vi "ComputeAreaUsingMoment.vi"(10 "Image In":T1) -> (1 "w_fy":dbl, 2 "w_fx":dbl, 4 "Y Centroid":sgl, 5 "X Centroid":sgl)   [LabVIEW 2018]
uses:
  <vilib>/vision/Image Controls.llb/IMAQ Image.ctl
  <vilib>/vision/NI_Vision_Development_Module.lvlib
panel:
  in  "File Path":path
  out "<xy>":dbl
  out "E(x,y)(x-xbar)(y-ybar)":dbl
  out "<y^2>":dbl
  out "E(x,y)(y-ybar)^2":dbl
  out "<x^2>":dbl
  out "E(x,y)(x-xbar)^2":dbl
  out "E(x,y)":dbl
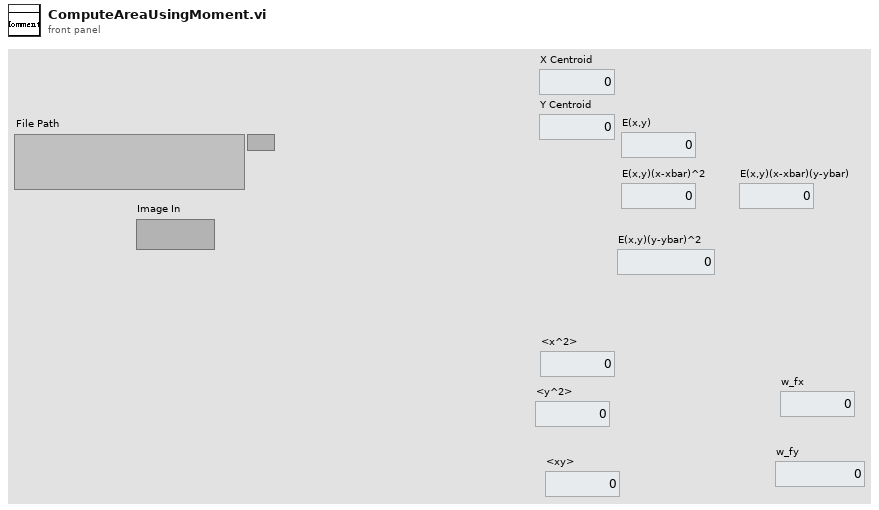
[diagram p1: front panel]
types:
  T1 = typedef "IMAQ Image.ctl" = refnum<image>
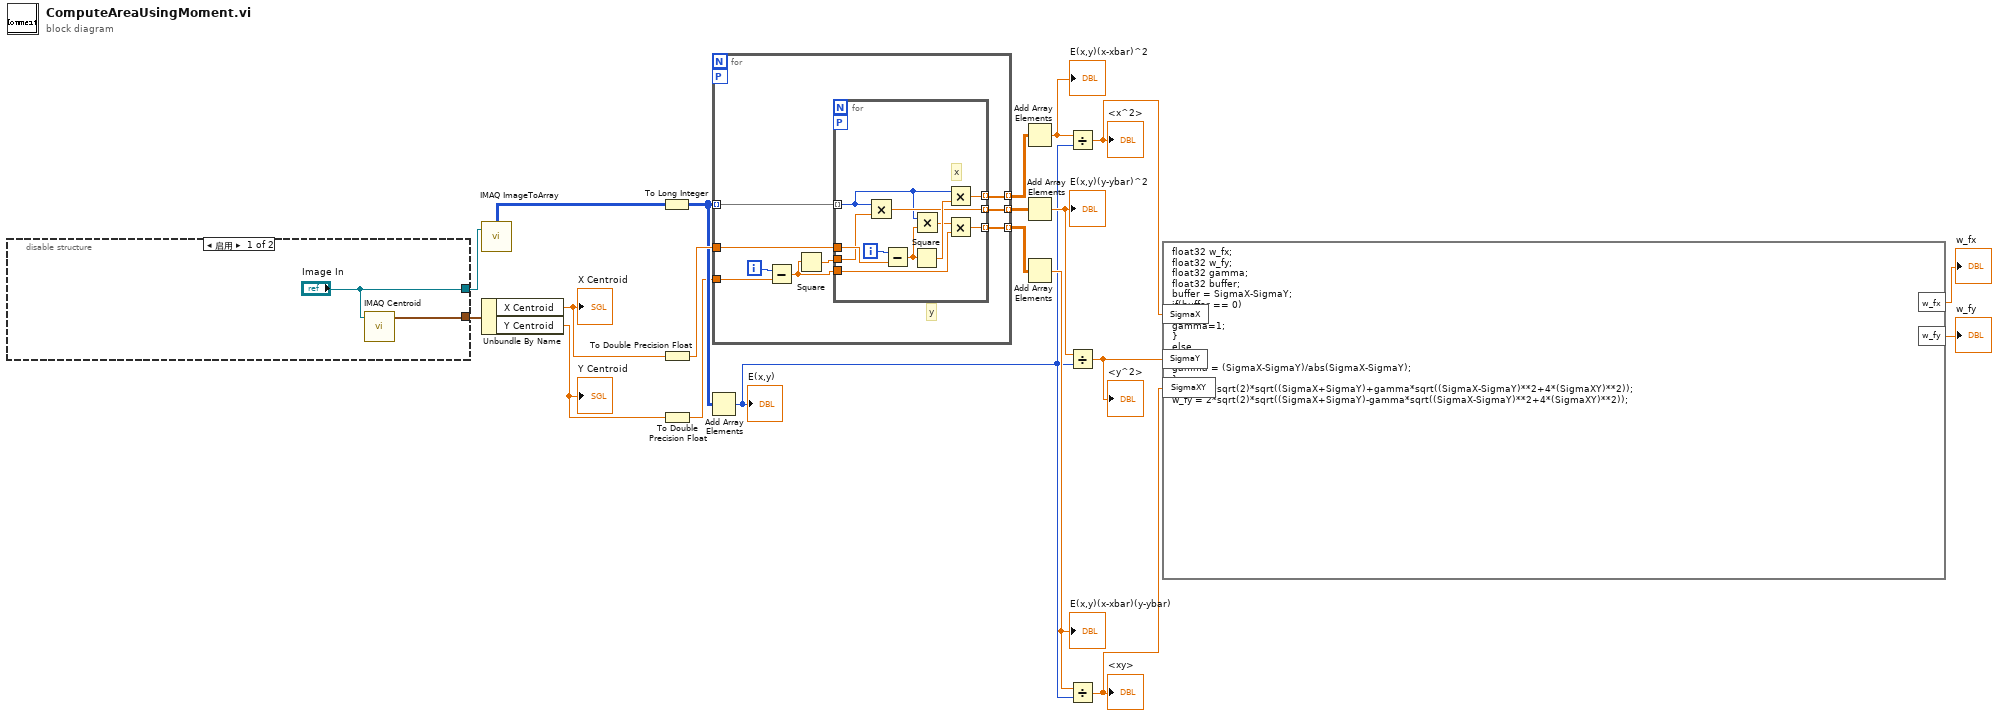
[diagram p0: block diagram]
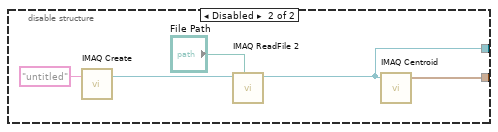
[diagram p2: hidden frame]
diagram:
  n1 = disable-structure shown="启用" {
    disable-tunnel: ["Image In" w24] -> w20
    disable-tunnel: [w21 w23] -> w1
    frame Enabled {
      n2 = call "IMAQ Centroid"("Image"="Image In") -> ("Centroid"=w21:cluster{"X Centroid":sgl, "Y Centroid":sgl})  [unwired: 3 in, 1 out]
    }
    frame Disabled {
      n3 = call "IMAQ Create"("Image Name"="untitled") -> ("New Image"=w27:T1)  [unwired: 4 in, 1 out]
      n4 = call "IMAQ ReadFile 2"("File Path"="File Path", "Image"=w27) -> ("Image Out"=w24:T1)  [unwired: 5 in, 4 out]
      n5 = call "IMAQ Centroid"("Image"=w24) -> ("Centroid"=w23:cluster{"X Centroid":sgl, "Y Centroid":sgl})  [unwired: 3 in, 1 out]
    }
  }
  n6 = call "IMAQ ImageToArray"("Image"=w20) -> ("Image Pixels (U8)"=w19:u8[][])  [unwired: 3 in, 4 out]
  n7 = Unbundle By Name(w1) -> ("X Centroid"=w18:sgl, "Y Centroid"=w14:sgl)
  "X Centroid" <- w18
  "Y Centroid" <- w14
  n8 = To Long Integer(number=w19) -> (32bit integer=w12:i32[][])
  n9 = To Double Precision Float(number=w18) -> (double precision float=w16:dbl)
  n10 = To Double Precision Float(number=w14) -> (double precision float=w11:dbl)
  n11 = Add Array Elements(numeric array=w12) -> (sum=w7:i32)
  "E(x,y)" <- w7
  n12 = for {
    tunnel: w12 -> [w36] mode=indexing
    workers-P: _ -> [_]
    tunnel: w16 -> [w35]
    tunnel: [w34] -> w17 mode=indexing
    tunnel: w11 -> [w33]
    tunnel: [w30] -> w10 mode=indexing
    tunnel: [w28] -> w9 mode=indexing
    i -> [w32]
    # "y"
    n13 = Subtract(x=w32, y=w33) -> (x-y=w29:dbl)
    n14 = Square(x=w29) -> (x^2=w31:dbl)
    n15 = for {
      tunnel: w36 -> [w41] mode=indexing
      workers-P: _ -> [_]
      tunnel: w35 -> [w47]
      tunnel: [w45] -> w34 mode=indexing
      tunnel: w31 -> [w43]
      tunnel: [w42] -> w30 mode=indexing
      tunnel: w29 -> [w38]
      tunnel: [w37] -> w28 mode=indexing
      i -> [w44]
      # "x"
      n16 = Multiply(x=w41, y=w43) -> (x*y=w42:dbl)
      n17 = Subtract(x=w44, y=w47) -> (x-y=w40:dbl)
      n18 = Square(x=w40) -> (x^2=w46:dbl)
      n19 = Multiply(x=w41, y=w40) -> (x*y=w39:dbl)
      n20 = Multiply(x=w41, y=w46) -> (x*y=w45:dbl)
      n21 = Multiply(x=w39, y=w38) -> (x*y=w37:dbl)
    }
  }
  n22 = Add Array Elements(numeric array=w17) -> (sum=w15:dbl)
  "E(x,y)(x-xbar)^2" <- w15
  n23 = Add Array Elements(numeric array=w10) -> (sum=w13:dbl)
  "E(x,y)(y-ybar)^2" <- w13
  n24 = Add Array Elements(numeric array=w9) -> (sum=w8:dbl)
  "E(x,y)(x-xbar)(y-ybar)" <- w8
  n25 = Divide(x=w15, y=w7) -> (x/y=w4:dbl)
  "<x^2>" <- w4
  n26 = Divide(x=w13, y=w7) -> (x/y=w5:dbl)
  "<y^2>" <- w5
  n27 = Divide(x=w8, y=w7) -> (x/y=w6:dbl)
  "<xy>" <- w6
  n28 = formula code="float32 w_fx;\nfloat32 w_fy;\nfloat32 gamma;\nfloat32 buffer;\nbuffer = SigmaX-SigmaY;\nif(buffer == 0)\n{\ngamma=1;\n}\nelse\n{\ngamma = (SigmaX-SigmaY)/abs(SigmaX-SigmaY);\n}\nw_fx = 2*sqrt(2)*sqrt((SigmaX+SigmaY)+gamma*sqrt((SigmaX-SigmaY)**2+4*(SigmaXY)**2));\nw_fy = 2*sqrt(2)*sqrt((SigmaX+SigmaY)-gamma*sqrt((SigmaX-SigmaY)**2+4*(SigmaXY)**2));"("SigmaX"=w4, "SigmaY"=w5, "SigmaXY"=w6) -> ("w_fx"=→"w_fx":sgl, "w_fy"=→"w_fy":sgl)
